vi "uEye_Binning_and_Subsampling.vi"() -> ()   [LabVIEW 2010]
uses:
  C:/Program Files (x86)/National Instruments/LabVIEW 2016/instr.lib/IDS/ueye.NET/uEyeDotNet.dll
  Program Files (x86)/National Instruments/LabVIEW 2016/instr.lib/IDS/ueye.NET/uEyeDotNet.dll
panel:
  out "Sensor Name":string
  out "Selected \nSubsampling Mode\nsupported":bool
  out "Selected \nBinning Mode \nsupported":bool
  in  "Vertical":i32(ring) items=["1x"=0, "2x"=1, "3x"=16, "4x"=4, "5x"=64, "6x"=256, "8x"=1024, "16x"=4096]
  in  "Horizontal":i32(ring) items=["1x"=0, "2x"=2, "3x"=32, "4x"=8, "5x"=128, "6x"=512, "8x"=2048, "16x"=8192]
  in  "Vertical":i32(ring) items=["1x"=0, "2x"=1, "3x"=16, "4x"=4, "5x"=64, "6x"=256, "8x"=1024, "16x"=4096]
  in  "Horizontal":i32(ring) items=["1x"=0, "2x"=2, "3x"=32, "4x"=8, "5x"=128, "6x"=512, "8x"=2048, "16x"=8192]
  out "Image":picture
  in  "Camera ID":i32 min=0 max=255
  out "Serial Number":string
  out "Height":i32=8
  out "Width":i32=8
  out "Bits/Pixel":i32=8
  out "Error Out":errorcluster caption="error"
  in  "Exit Camera":bool
  in  "Init Camera":bool
  # "Binning"
  # "Subsampling"
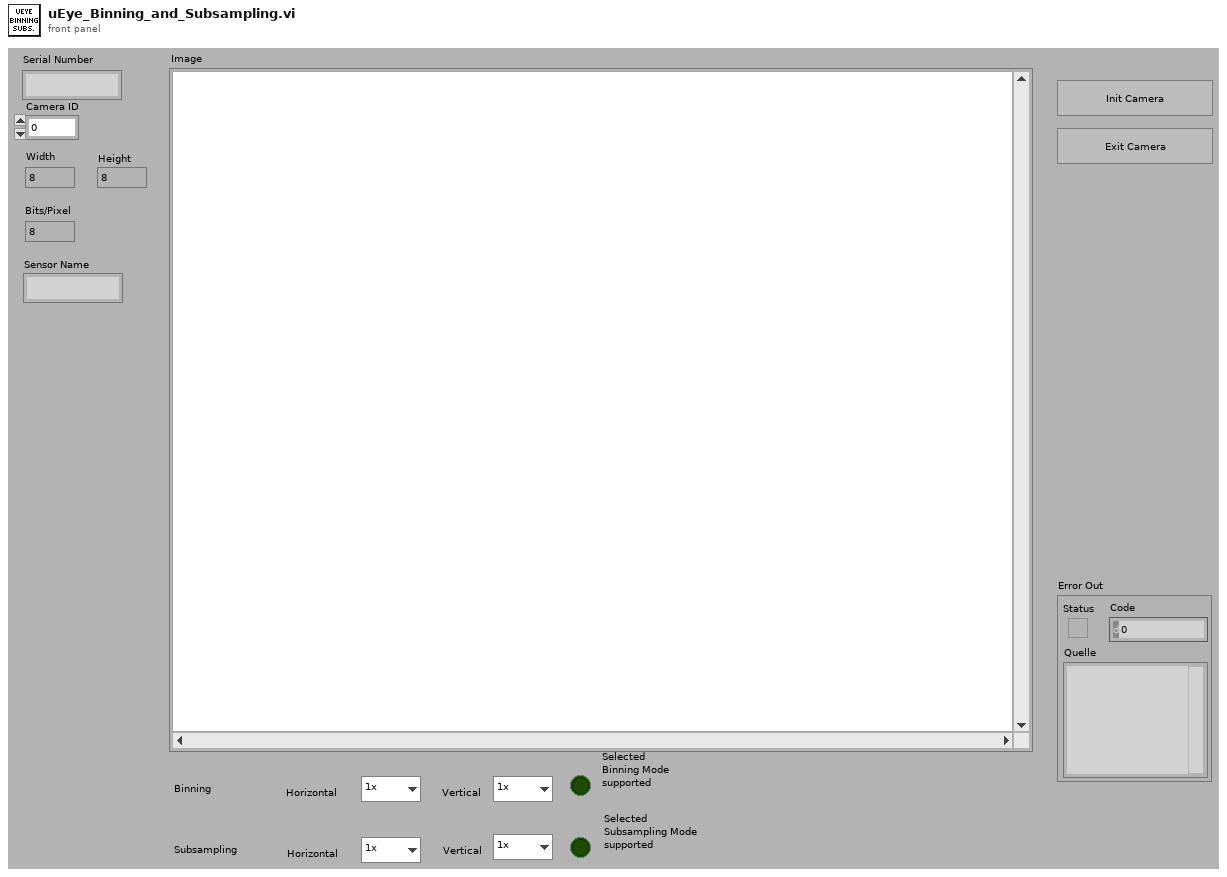
[diagram p1: front panel]
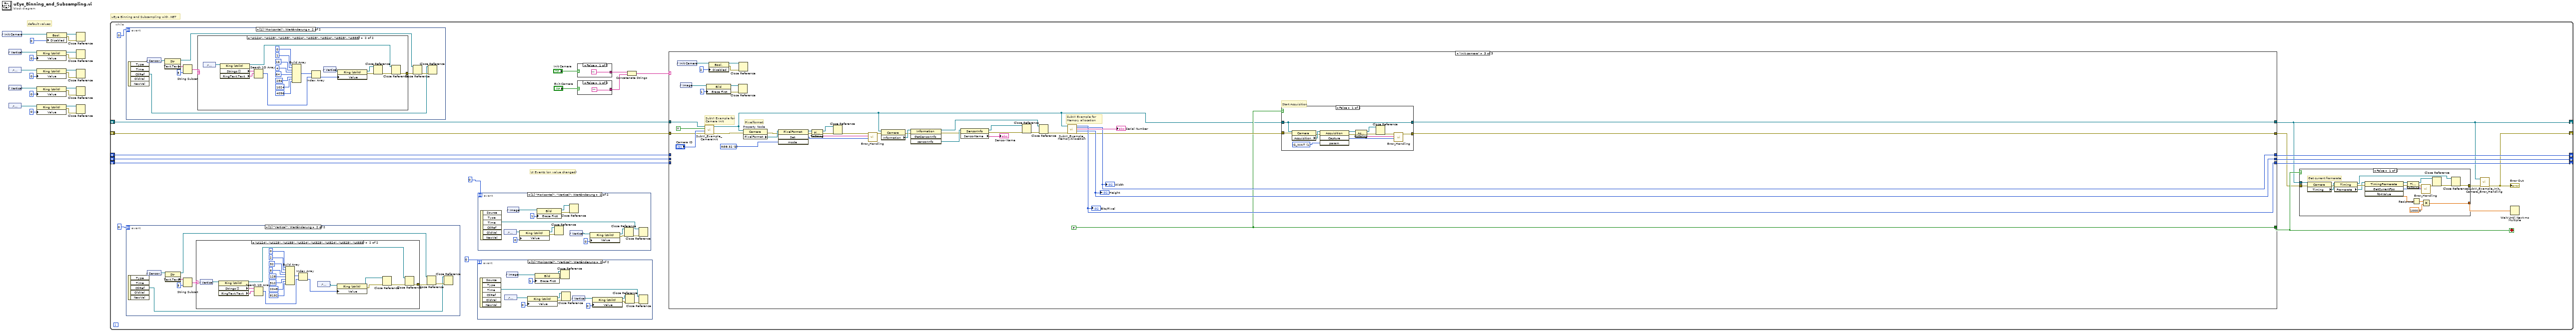
[diagram p0: block diagram]
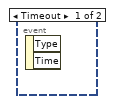
[diagram p2: hidden frame]
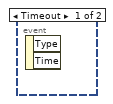
[diagram p4: hidden frame]
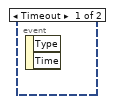
[diagram p6: hidden frame]
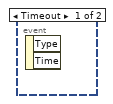
[diagram p7: hidden frame]
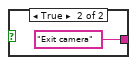
[diagram p8: hidden frame]
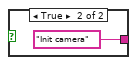
[diagram p9: hidden frame]
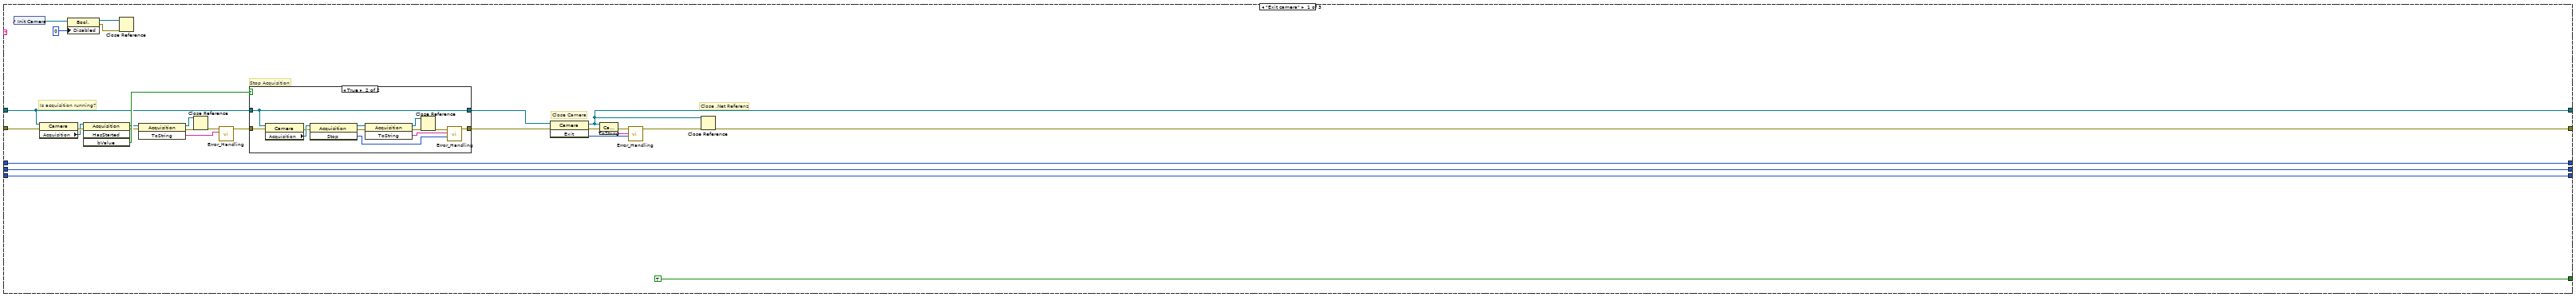
[diagram p10: hidden frame]
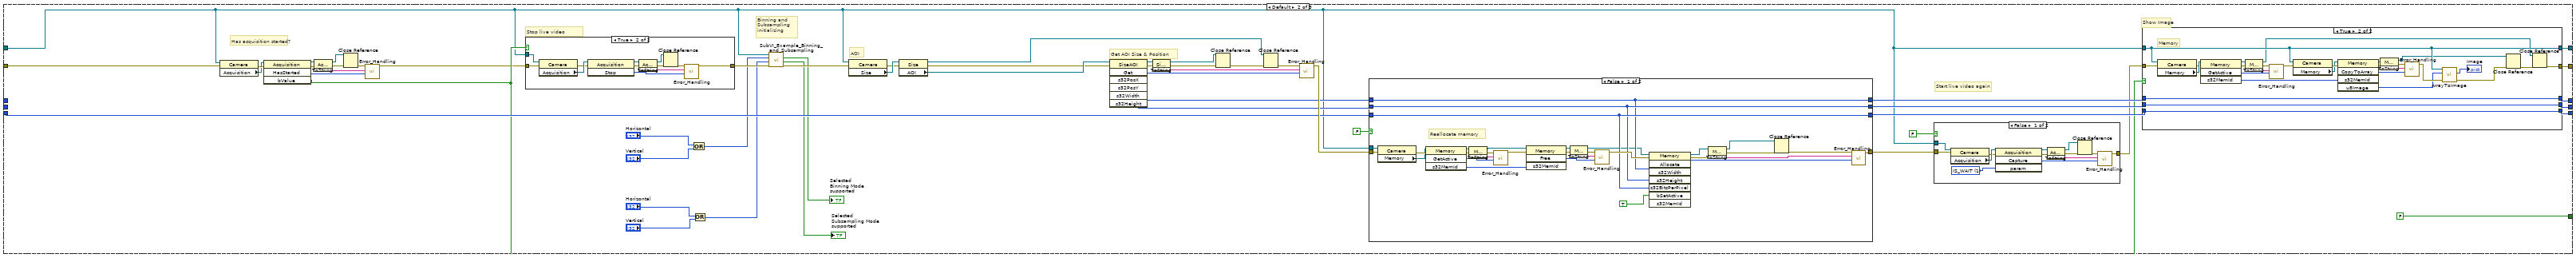
[diagram p12: hidden frame]
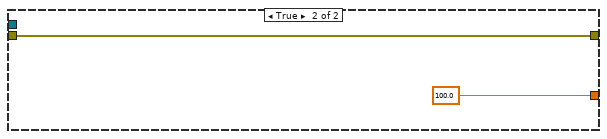
[diagram p18: hidden frame]
diagram:
  # "default values"
  # "uEye Binning and Subsampling with .NET"
  n1 = control-ref of="Init Camera"() -> (w19:refnum<vi>)
  n2 = control-ref of="Vertical"() -> (w11:refnum<vi>)
  n3 = control-ref of="Horizontal"() -> (w12:refnum<vi>)
  n4 = control-ref of="Vertical"() -> (w13:refnum<vi>)
  n5 = control-ref of="Horizontal"() -> (w14:refnum<vi>)
  n6 = property class="Ring (strikt)"(reference=w11, "Value"=0) -> (reference out=w8:refnum<vi>, error out=w7:errorcluster)  [unwired: 1 in]
  n7 = property class="Ring (strikt)"(reference=w12, "Value"=0) -> (reference out=w6:refnum<vi>, error out=w5:errorcluster)  [unwired: 1 in]
  n8 = property class="Ring (strikt)"(reference=w13, "Value"=0) -> (reference out=w4:refnum<vi>, error out=w3:errorcluster)  [unwired: 1 in]
  n9 = property class="Ring (strikt)"(reference=w14, "Value"=0) -> (reference out=w2:refnum<vi>, error out=w1:errorcluster)  [unwired: 1 in]
  n10 = property class="Bool."(reference=w19, "Disabled"=u8 0 ("Deaktiviert")) -> (reference out=w10:refnum<vi>, error out=w9:errorcluster)  [unwired: 1 in]
  n11 = Close Reference(reference=w10, error in (no error)=w9) -> ()  [unwired: 1 out]
  n12 = Close Reference(reference=w8, error in (no error)=w7) -> ()  [unwired: 1 out]
  n13 = Close Reference(reference=w6, error in (no error)=w5) -> ()  [unwired: 1 out]
  n14 = Close Reference(reference=w4, error in (no error)=w3) -> ()  [unwired: 1 out]
  n15 = Close Reference(reference=w2, error in (no error)=w1) -> ()  [unwired: 1 out]
  n16 = while {
    shift-right: [w28] -> _
    shift-left: _ -> [w38]
    shift-right: [w27] -> _
    shift-left: _ -> [w21]
    shift-right: [w35] -> _
    shift-left: _ -> [w34]
    shift-right: [w37] -> _
    shift-left: _ -> [w33]
    shift-right: [w36] -> _
    shift-left: _ -> [w32]
    stop <- w31 stop-if-true
    # "UI Events (on value changed)"
    n17 = event shown="[1] \"Horizontal\": Wertänderung" {
      selector: _ -> [_ _]
      dyn-events: _ -> [_ _]
      timeout: 0 -> [_ _]
      event Timeout {
        n18 = event-data() -> ()  [unwired: 1 in, 2 out]
      }
      event "Horizontal": Value Change {
        n19 = event-data() -> ("CtlRef"=w72:refnum<vi>)  [unwired: 1 in, 4 out]
        n20 = control-ref of="Sensor Name"() -> (w79:refnum<vi>)
        n21 = property class="Str"(reference=w79) -> (reference out=w74:refnum<vi>, "Text.Text"=w78:string)  [unwired: 1 in, 1 out]
        n22 = String Subset(string=w78, length (rest)=5 ("length (rest)")) -> (substring=w76:string)  [unwired: 1 in]
        n23 = case shown="\"UI124\", \"UI125\", \"UI155\", \"UI324\", \"UI325\", \"UI524\", \"UI525\", \"UI555\"" w76 {
          tunnel: [_ w80] -> w75
          frame "False", Default {
          }
          frame "UI124", "UI125", "UI155", "UI324", "UI325", "UI524", "UI525", "UI555" {
            n24 = control-ref of="Horizontal"() -> (w99:refnum<vi>)
            n25 = property class="Ring (strikt)"(reference=w99) -> (reference out=w81:refnum<vi>, "Strings []"=w97:string[], "RingText.Text"=w96:string)  [unwired: 1 in, 1 out]
            n26 = Search 1D Array(1D array=w97, element=w96) -> (index of element=w86:i32)  [unwired: 1 in]
            n27 = Build Array(0, 1, 16, 4, 64, 256, 1024, 4096) -> (w95:i32[])
            n28 = Index Array(array=w95, index=w86) -> (element=w85:i32)
            n29 = control-ref of="Vertical"() -> (w98:refnum<vi>)
            n30 = property class="Ring (strikt)"(reference=w98, "Value"=w85) -> (reference out=w83:refnum<vi>, error out=w84:errorcluster)  [unwired: 1 in]
            n31 = Close Reference(reference=w83, error in (no error)=w84) -> (error out=w82:errorcluster)
            n32 = Close Reference(reference=w81, error in (no error)=w82) -> (error out=w80:errorcluster)
          }
        }
        n33 = Close Reference(reference=w74, error in (no error)=w75) -> (error out=w73:errorcluster)
        n34 = Close Reference(reference=w72, error in (no error)=w73) -> ()  [unwired: 1 out]
      }
    }
    n35 = event shown="[1] \"Vertical\": Wertänderung" {
      selector: _ -> [_ _]
      dyn-events: _ -> [_ _]
      timeout: 0 -> [_ _]
      event Timeout {
        n36 = event-data() -> ()  [unwired: 1 in, 2 out]
      }
      event "Vertical": Value Change {
        n37 = event-data() -> ("CtlRef"=w44:refnum<vi>)  [unwired: 1 in, 4 out]
        n38 = control-ref of="Sensor Name"() -> (w49:refnum<vi>)
        n39 = property class="Str"(reference=w49) -> (reference out=w45:refnum<vi>, "Text.Text"=w51:string)  [unwired: 1 in, 1 out]
        n40 = String Subset(string=w51, length (rest)=5 ("length (rest)")) -> (substring=w48:string)  [unwired: 1 in]
        n41 = case shown="\"UI124\", \"UI125\", \"UI155\", \"UI324\", \"UI325\", \"UI524\", \"UI525\", \"UI555\"" w48 {
          tunnel: [_ w56] -> w46
          frame "False", Default {
          }
          frame "UI124", "UI125", "UI155", "UI324", "UI325", "UI524", "UI525", "UI555" {
            n42 = control-ref of="Vertical"() -> (w70:refnum<vi>)
            n43 = property class="Ring (strikt)"(reference=w70) -> (reference out=w55:refnum<vi>, "Strings []"=w69:string[], "RingText.Text"=w68:string)  [unwired: 1 in, 1 out]
            n44 = Search 1D Array(1D array=w69, element=w68) -> (index of element=w58:i32)  [unwired: 1 in]
            n45 = Build Array(0, 2, 32, 8, 128, 512, 2048, 8192) -> (w59:i32[])
            n46 = Index Array(array=w59, index=w58) -> (element=w57:i32)
            n47 = control-ref of="Horizontal"() -> (w71:refnum<vi>)
            n48 = property class="Ring (strikt)"(reference=w71, "Value"=w57) -> (reference out=w52:refnum<vi>, error out=w53:errorcluster)  [unwired: 1 in]
            n49 = Close Reference(reference=w52, error in (no error)=w53) -> (error out=w54:errorcluster)
            n50 = Close Reference(reference=w55, error in (no error)=w54) -> (error out=w56:errorcluster)
          }
        }
        n51 = Close Reference(reference=w45, error in (no error)=w46) -> (error out=w47:errorcluster)
        n52 = Close Reference(reference=w44, error in (no error)=w47) -> ()  [unwired: 1 out]
      }
    }
    n53 = event shown="[1] \"Horizontal\", \"Vertical\": Wertänderung" {
      selector: _ -> [_ _]
      dyn-events: _ -> [_ _]
      timeout: 0 -> [_ _]
      event Timeout {
        n54 = event-data() -> ()  [unwired: 1 in, 2 out]
      }
      event "Horizontal", "Vertical": Value Change {
        n55 = event-data() -> ("CtlRef"=w100:refnum<vi>)  [unwired: 1 in, 5 out]
        n56 = control-ref of="Horizontal"() -> (w110:refnum<vi>)
        n57 = control-ref of="Image"() -> (w112:refnum<vi>)
        n58 = property class="Ring (strikt)"(reference=w110, "Value"=0) -> (reference out=w104:refnum<vi>, error out=w105:errorcluster)  [unwired: 1 in]
        n59 = property class="Bild"(reference=w112, "Erase First"=u8 1 ("Zuerst löschen")) -> (reference out=w106:refnum<vi>, error out=w107:errorcluster)  [unwired: 1 in]
        n60 = Close Reference(reference=w106, error in (no error)=w107) -> ()  [unwired: 1 out]
        n61 = Close Reference(reference=w104, error in (no error)=w105) -> ()  [unwired: 1 out]
        n62 = control-ref of="Vertical"() -> (w108:refnum<vi>)
        n63 = property class="Ring (strikt)"(reference=w108, "Value"=0) -> (reference out=w102:refnum<vi>, error out=w103:errorcluster)  [unwired: 1 in]
        n64 = Close Reference(reference=w102, error in (no error)=w103) -> (error out=w101:errorcluster)
        n65 = Close Reference(reference=w100, error in (no error)=w101) -> ()  [unwired: 1 out]
      }
    }
    n66 = event shown="[1] \"Horizontal\", \"Vertical\": Wertänderung" {
      selector: _ -> [_ _]
      dyn-events: _ -> [_ _]
      timeout: 0 -> [_ _]
      event Timeout {
        n67 = event-data() -> ()  [unwired: 1 in, 2 out]
      }
      event "Horizontal", "Vertical": Value Change {
        n68 = event-data() -> ("CtlRef"=w114:refnum<vi>)  [unwired: 1 in, 5 out]
        n69 = control-ref of="Horizontal"() -> (w125:refnum<vi>)
        n70 = control-ref of="Image"() -> (w126:refnum<vi>)
        n71 = property class="Ring (strikt)"(reference=w125, "Value"=0) -> (reference out=w119:refnum<vi>, error out=w118:errorcluster)  [unwired: 1 in]
        n72 = property class="Bild"(reference=w126, "Erase First"=u8 1 ("Zuerst löschen")) -> (reference out=w121:refnum<vi>, error out=w120:errorcluster)  [unwired: 1 in]
        n73 = Close Reference(reference=w119, error in (no error)=w118) -> ()  [unwired: 1 out]
        n74 = Close Reference(reference=w121, error in (no error)=w120) -> ()  [unwired: 1 out]
        n75 = control-ref of="Vertical"() -> (w122:refnum<vi>)
        n76 = property class="Ring (strikt)"(reference=w122, "Value"=0) -> (reference out=w116:refnum<vi>, error out=w117:errorcluster)  [unwired: 1 in]
        n77 = Close Reference(reference=w116, error in (no error)=w117) -> (error out=w115:errorcluster)
        n78 = Close Reference(reference=w114, error in (no error)=w115) -> ()  [unwired: 1 out]
      }
    }
    n79 = case shown="False" "Init Camera" {
      tunnel: ["" "Init camera"] -> w42
      frame False {
      }
      frame True {
      }
    }
    n80 = case shown="False" "Exit Camera" {
      tunnel: ["" "Exit camera"] -> w39
      frame False {
      }
      frame True {
      }
    }
    n81 = Concatenate Strings(w42, w39) -> (w41:string)
    n82 = case shown="\"Init camera\"" w41 {
      tunnel: w21 -> [w141 w190 w358]
      tunnel: w38 -> [w142 w183 w357]
      tunnel: [w153 w217 w348] -> w27
      tunnel: [w154 w216 w347] -> w30
      tunnel: [w152 w220 w351] -> w35
      tunnel: [w151 w219 w352] -> w37
      tunnel: [w150 w218 w353] -> w36
      tunnel: w34 -> [w152 _ _]
      tunnel: w33 -> [w151 _ _]
      tunnel: w32 -> [w150 w206 _]
      tunnel: [TRUE FALSE w349] -> w31
      frame "Exit camera" {
        # "Close .Net Referenz"
        # "Is acquisition running?"
        # "Stop Acquisition"
        # "Close Camera"
        n83 = control-ref of="Init Camera"() -> (w137:refnum<vi>)
        n84 = property class="Camera"(reference=w141, error in=w142) -> (error out=w149:errorcluster, "Acquisition"=w148:refnum<k24>)  [unwired: 1 out]
        n85 = property class="Bool."(reference=w137, "Disabled"=u8 0 ("Deaktiviert")) -> (reference out=w132:refnum<vi>, error out=w133:errorcluster)  [unwired: 1 in]
        n86 = invoke class="Acquisition" method="HasStarted"(reference=w148, error in=w149) -> (reference out=w143:refnum<k24>, error out=w145:errorcluster, "bValue"=w147:bool)  [unwired: 2 in, 1 out]
        n87 = Close Reference(reference=w132, error in (no error)=w133) -> ()  [unwired: 1 out]
        n88 = invoke class="Acquisition" method="ToString"(reference=w143, error in=w145) -> (reference out=w134:refnum<k24>, error out=w136:errorcluster, "ToString"=w144:string)  [unwired: 1 in]
        n89 = Close Reference(reference=w134, error in (no error)=w136) -> (error out=w135:errorcluster)
        n90 = call "Error_Handling.vi"("Error String"=w144, "Error In"=w135) -> ("Error Out"=w146:errorcluster)  [unwired: 9 in]
        n91 = case shown="True" w147 {
          tunnel: [w162 w173] -> w139
          tunnel: w146 -> [w162 w174]
          tunnel: w141 -> [w161 w166]
          tunnel: [w161 w166] -> w140
          frame False {
          }
          frame True {
            n92 = property class="Camera"(reference=w166, error in=w174) -> (error out=w170:errorcluster, "Acquisition"=w171:refnum<k24>)  [unwired: 1 out]
            n93 = invoke class="Acquisition" method="Stop"(reference=w171, error in=w170) -> (reference out=w168:refnum<k24>, error out=w169:errorcluster, "Stop"=w167:i32)  [unwired: 1 in]
            n94 = invoke class="Acquisition" method="ToString"(reference=w168, error in=w169) -> (reference out=w163:refnum<k24>, error out=w165:errorcluster, "ToString"=w172:string)  [unwired: 1 in]
            n95 = Close Reference(reference=w163, error in (no error)=w165) -> (error out=w164:errorcluster)
            n96 = call "Error_Handling.vi"("Error Code"=w167, "Error String"=w172, "Error In"=w164) -> ("Error Out"=w173:errorcluster)  [unwired: 8 in]
          }
        }
        n97 = invoke class="Camera" method="Exit"(reference=w140, error in=w139) -> (reference out=w153:refnum<k24>, error out=w157:errorcluster, "Exit"=w156:i32)  [unwired: 1 in]
        n98 = invoke class="Camera" method="ToString"(reference=w153, error in=w157) -> (error out=w158:errorcluster, "ToString"=w159:string)  [unwired: 1 in, 1 out]
        n99 = call "Error_Handling.vi"("Error Code"=w156, "Error String"=w159, "Error In"=w158) -> ("Error Out"=w155:errorcluster)  [unwired: 8 in]
        n100 = Close Reference ("Close Referenz")(reference=w153, error in (no error)=w155) -> (error out=w154:errorcluster)
      }
      frame Default {
        # "Binning and Subsampling initializing"
        # "Start live video again"
        # "Stop live video"
        # "Get AOI Size & Position"
        # "AOI"
        # "Has acquisition started?"
        # "Show Image"
        n101 = property class="Camera"(reference=w190, error in=w183) -> (error out=w226:errorcluster, "Acquisition"=w225:refnum<k24>)  [unwired: 1 out]
        n102 = invoke class="Acquisition" method="HasStarted"(reference=w225, error in=w226) -> (reference out=w223:refnum<k24>, error out=w222:errorcluster, "HasStarted"=w221:i32, "bValue"=w202:bool)  [unwired: 2 in]
        n103 = invoke class="Acquisition" method="ToString"(reference=w223, error in=w222) -> (reference out=w175:refnum<k24>, error out=w177:errorcluster, "ToString"=w224:string)  [unwired: 1 in]
        n104 = Close Reference(reference=w175, error in (no error)=w177) -> (error out=w176:errorcluster)
        n105 = call "Error_Handling.vi"("Error Code"=w221, "Error String"=w224, "Error In"=w176) -> ("Error Out"=w185:errorcluster)  [unwired: 8 in]
        n106 = case shown="True" w202 {
          tunnel: [w228 w240] -> w192
          tunnel: w190 -> [_ w234]
          tunnel: w185 -> [w228 w233]
          frame False {
          }
          frame True {
            n107 = property class="Camera"(reference=w234, error in=w233) -> (error out=w232:errorcluster, "Acquisition"=w238:refnum<k24>)  [unwired: 1 out]
            n108 = invoke class="Acquisition" method="Stop"(reference=w238, error in=w232) -> (reference out=w236:refnum<k24>, error out=w237:errorcluster, "Stop"=w235:i32)  [unwired: 1 in]
            n109 = invoke class="Acquisition" method="ToString"(reference=w236, error in=w237) -> (reference out=w229:refnum<k24>, error out=w231:errorcluster, "ToString"=w239:string)  [unwired: 1 in]
            n110 = Close Reference(reference=w229, error in (no error)=w231) -> (error out=w230:errorcluster)
            n111 = call "Error_Handling.vi"("Error Code"=w235, "Error String"=w239, "Error In"=w230) -> ("Error Out"=w240:errorcluster)  [unwired: 8 in]
          }
        }
        n112 = Or(x="Horizontal", y="Vertical") -> (x .or. y?=w189:i32)
        n113 = Or(x="Horizontal", y="Vertical") -> (x .or. y?=w188:i32)
        n114 = call "SubVI_Example_Binning_and_Subsampling.vi"("Error In"=w192, "Subsampling Mode"=w188, "Binning Mode"=w189, ".NET (Reference)"=w190) -> ("Error Out"=w191:errorcluster, "Subsampling mode supported"=→"Selected \nSubsampling Mode\nsupported":bool, "Binning mode supported"=→"Selected \nBinning Mode \nsupported":bool)  [unwired: 5 in]
        n115 = property class="Camera"(reference=w190, error in=w191) -> (error out=w214:errorcluster, "Size"=w215:refnum<k24>)  [unwired: 1 out]
        n116 = property class="Size"(reference=w215, error in=w214) -> (reference out=w178:refnum<k24>, error out=w184:errorcluster, "AOI"=w193:refnum<k24>)
        n117 = invoke class="SizeAOI" method="Get"(reference=w193, error in=w184) -> (reference out=w212:refnum<k24>, error out=w211:errorcluster, "Get"=w210:i32, "s32Width"=w208:i32, "s32Height"=w207:i32)  [unwired: 5 in, 2 out]
        n118 = invoke class="SizeAOI" method="ToString"(reference=w212, error in=w211) -> (reference out=w181:refnum<k24>, error out=w182:errorcluster, "ToString"=w213:string)  [unwired: 1 in]
        n119 = Close Reference(reference=w181, error in (no error)=w182) -> (error out=w180:errorcluster)
        n120 = Close Reference(reference=w178, error in (no error)=w180) -> (error out=w179:errorcluster)
        n121 = call "Error_Handling.vi"("Error Code"=w210, "Error String"=w213, "Error In"=w179) -> ("Error Out"=w209:errorcluster)  [unwired: 8 in]
        n122 = case shown="False" FALSE {
          tunnel: w209 -> [w266 w286]
          tunnel: w208 -> [w262 w289]
          tunnel: w207 -> [w263 w288]
          tunnel: w206 -> [w264 w287]
          tunnel: [w265 w286] -> w201
          tunnel: [w264 w287] -> w205
          tunnel: [w263 w288] -> w204
          tunnel: [w262 w289] -> w203
          tunnel: w190 -> [w261 _]
          frame False {
            # "Reallocate memory"
            n123 = property class="Camera"(reference=w261, error in=w266) -> (error out=w268:errorcluster, "Memory"=w259:refnum<k24>)  [unwired: 1 out]
            n124 = invoke class="Memory" method="GetActive"(reference=w259, error in=w268) -> (reference out=w273:refnum<k24>, error out=w272:errorcluster, "GetActive"=w271:i32, "s32MemId"=w270:i32)  [unwired: 2 in]
            n125 = invoke class="Memory" method="ToString"(reference=w273, error in=w272) -> (reference out=w258:refnum<k24>, error out=w274:errorcluster, "ToString"=w275:string)  [unwired: 1 in]
            n126 = call "Error_Handling.vi"("Error Code"=w271, "Error String"=w275, "Error In"=w274) -> ("Error Out"=w269:errorcluster)  [unwired: 8 in]
            n127 = invoke class="Memory" method="Free"(reference=w258, error in=w269, "s32MemId"=w270) -> (reference out=w278:refnum<k24>, error out=w277:errorcluster, "Free"=w276:i32)  [unwired: 1 in, 1 out]
            n128 = invoke class="Memory" method="ToString"(reference=w278, error in=w277) -> (reference out=w255:refnum<k24>, error out=w279:errorcluster, "ToString"=w280:string)  [unwired: 1 in]
            n129 = call "Error_Handling.vi"("Error Code"=w276, "Error String"=w280, "Error In"=w279) -> ("Error Out"=w267:errorcluster)  [unwired: 8 in]
            n130 = invoke class="Memory" method="Allocate"(reference=w255, error in=w267, "s32Width"=w262, "s32Height"=w263, "s32BitsPerPixel"=w264, "bSetActive"=TRUE) -> (reference out=w284:refnum<k24>, error out=w283:errorcluster, "Allocate"=w282:i32)  [unwired: 2 in, 5 out]
            n131 = invoke class="Memory" method="ToString"(reference=w284, error in=w283) -> (reference out=w256:refnum<k24>, error out=w257:errorcluster, "ToString"=w285:string)  [unwired: 1 in]
            n132 = Close Reference(reference=w256, error in (no error)=w257) -> (error out=w260:errorcluster)
            n133 = call "Error_Handling.vi"("Error Code"=w282, "Error String"=w285, "Error In"=w260) -> ("Error Out"=w265:errorcluster)  [unwired: 8 in]
          }
          frame True {
          }
        }
        n134 = case shown="False" FALSE {
          tunnel: [w246 w254] -> w199
          tunnel: w201 -> [w251 w254]
          tunnel: w190 -> [w250 _]
          frame False {
            w244 = 1 items=["IS_DONT_WAIT", "IS_WAIT"] ("Wait")
            n135 = property class="Camera"(reference=w250, error in=w251) -> (error out=w252:errorcluster, "Acquisition"=w253:refnum<k24>)  [unwired: 1 out]
            n136 = invoke class="Acquisition" method="Capture"(reference=w253, error in=w252, "param"=w244) -> (reference out=w247:refnum<k24>, error out=w248:errorcluster, "Capture"=w245:i32)  [unwired: 1 in, 1 out]
            n137 = invoke class="Acquisition" method="ToString"(reference=w247, error in=w248) -> (reference out=w241:refnum<k24>, error out=w243:errorcluster, "ToString"=w249:string)  [unwired: 1 in]
            n138 = Close Reference(reference=w241, error in (no error)=w243) -> (error out=w242:errorcluster)
            n139 = call "Error_Handling.vi"("Error Code"=w245, "Error String"=w249, "Error In"=w242) -> ("Error Out"=w246:errorcluster)  [unwired: 8 in]
          }
          frame True {
          }
        }
        n140 = case shown="True" w202 {
          tunnel: [w294 w299] -> w216
          tunnel: w199 -> [w294 w304]
          tunnel: w190 -> [w293 w300]
          tunnel: [w293 w300] -> w217
          tunnel: w203 -> [w292 w307]
          tunnel: w204 -> [w291 w306]
          tunnel: w205 -> [w290 w305]
          tunnel: [w292 w307] -> w220
          tunnel: [w291 w306] -> w219
          tunnel: [w290 w305] -> w218
          frame False {
          }
          frame True {
            # "Memory"
            n141 = property class="Camera"(reference=w300, error in=w304) -> (error out=w309:errorcluster, "Memory"=w310:refnum<k24>)  [unwired: 1 out]
            n142 = invoke class="Memory" method="GetActive"(reference=w310, error in=w309) -> (reference out=w316:refnum<k24>, error out=w315:errorcluster, "GetActive"=w317:i32, "s32MemId"=w308:i32)  [unwired: 2 in]
            n143 = invoke class="Memory" method="ToString"(reference=w316, error in=w315) -> (reference out=w298:refnum<k24>, error out=w313:errorcluster, "ToString"=w314:string)  [unwired: 1 in]
            n144 = call "Error_Handling.vi"("Error Code"=w317, "Error String"=w314, "Error In"=w313) -> ("Error Out"=w318:errorcluster)  [unwired: 8 in]
            n145 = property class="Camera"(reference=w300, error in=w318) -> (error out=w312:errorcluster, "Memory"=w311:refnum<k24>)  [unwired: 1 out]
            n146 = invoke class="Memory" method="CopyToArray"(reference=w311, error in=w312, "s32MemId"=w308) -> (reference out=w321:refnum<k24>, error out=w322:errorcluster, "CopyToArray"=w323:i32, "u8Image"=w301:u8[])  [unwired: 2 in, 1 out]
            n147 = invoke class="Memory" method="ToString"(reference=w321, error in=w322) -> (reference out=w295:refnum<k24>, error out=w319:errorcluster, "ToString"=w320:string)  [unwired: 1 in]
            n148 = call "Error_Handling.vi"("Error Code"=w323, "Error String"=w320, "Error In"=w319) -> ("Error Out"=w302:errorcluster)  [unwired: 8 in]
            n149 = call "ArrayToImage.vi"("Error In"=w302, "InArray"=w301, ".NET (Reference)"=w300) -> ("Error Out"=w296:errorcluster, "Image"=→"Image":picture)  [unwired: 7 in]
            n150 = Close Reference(reference=w295, error in (no error)=w296) -> (error out=w297:errorcluster)
            n151 = Close Reference(reference=w298, error in (no error)=w297) -> (error out=w299:errorcluster)
          }
        }
      }
      frame "Init camera" {
        w349 = FALSE
        w366 = 0 items=["RGB 32"=0, "RGB 24"=1, "Y8 Monochrom"=6] ("Mode")
        # "Start Acquisition"
        # "SubVI Example for \nMemory allocation"
        # "SubVI Example for \nCamera Init"
        # "Pixelformat"
        n152 = control-ref of="Init Camera"() -> (w346:refnum<vi>)
        n153 = control-ref of="Image"() -> (w343:refnum<vi>)
        n154 = call "SubVI_Example_CameraInit.vi"("Error In"=w357, "Camera ID"="Camera ID", "Init Camera Flag"=TRUE, ".NET (Reference)"=w358) -> ("Error Out"=w363:errorcluster, ".NET (Reference)"=w340:refnum<k24>)  [unwired: 6 in]
        n155 = property class="Bild"(reference=w343, "Erase First"=u8 1 ("Zuerst löschen")) -> (reference out=w325:refnum<vi>, error out=w326:errorcluster)  [unwired: 1 in]
        n156 = property class="Bool."(reference=w346, "Disabled"=u8 2 ("Deaktiviert")) -> (reference out=w324:refnum<vi>, error out=w327:errorcluster)  [unwired: 1 in]
        n157 = Close Reference(reference=w325, error in (no error)=w326) -> ()  [unwired: 1 out]
        n158 = Close Reference(reference=w324, error in (no error)=w327) -> ()  [unwired: 1 out]
        n159 = property on="Property Node" class="Camera"(reference=w340, error in=w363) -> (error out=w364:errorcluster, "PixelFormat"=w365:refnum<k24>)  [unwired: 1 out]
        n160 = invoke class="PixelFormat" method="Set"(reference=w365, error in=w364, "mode"=w366) -> (reference out=w361:refnum<k24>, error out=w355:errorcluster, "Set"=w360:i32)  [unwired: 1 in, 1 out]
        n161 = invoke class="PixelFormat" method="ToString"(reference=w361, error in=w355) -> (reference out=w333:refnum<k24>, error out=w335:errorcluster, "ToString"=w362:string)  [unwired: 1 in]
        n162 = Close Reference(reference=w333, error in (no error)=w335) -> (error out=w334:errorcluster)
        n163 = call "Error_Handling.vi"("Error Code"=w360, "Error String"=w362, "Error In"=w334) -> ("Error Out"=w341:errorcluster)  [unwired: 8 in]
        n164 = property class="Camera"(reference=w340, error in=w341) -> (error out=w339:errorcluster, "Information"=w342:refnum<k24>)  [unwired: 1 out]
        n165 = invoke class="Information" method="GetSensorInfo"(reference=w342, error in=w339) -> (reference out=w328:refnum<k24>, error out=w337:errorcluster, "sensorInfo"=w338:refnum<k24>)  [unwired: 2 in, 1 out]
        n166 = property class="SensorInfo"(reference=w338, error in=w337) -> (reference out=w331:refnum<k24>, error out=w332:errorcluster, "SensorName"=→"Sensor Name":string)
        n167 = Close Reference(reference=w331, error in (no error)=w332) -> (error out=w330:errorcluster)
        n168 = Close Reference(reference=w328, error in (no error)=w330) -> (error out=w329:errorcluster)
        n169 = call "SubVI_Example_MemoryAllocation.vi"(".NET (Reference)"=w340, "Error In"=w329) -> ("Bits/Pixel 2"=w353:i32, "Width"=w351:i32, "Serial Number"=→"Serial Number":string, "Height"=w352:i32, "Error Out"=w350:errorcluster)  [unwired: 13 in]
        "Bits/Pixel" <- w353
        "Width" <- w351
        "Height" <- w352
        n170 = case shown="False" w349 {
          tunnel: [w372 w381] -> w347
          tunnel: w350 -> [w377 w381]
          tunnel: w340 -> [w376 w380]
          tunnel: [w376 w380] -> w348
          frame False {
            w370 = 1 items=["IS_DONT_WAIT", "IS_WAIT"] ("Wait")
            n171 = property class="Camera"(reference=w376, error in=w377) -> (error out=w378:errorcluster, "Acquisition"=w379:refnum<k24>)  [unwired: 1 out]
            n172 = invoke class="Acquisition" method="Capture"(reference=w379, error in=w378, "param"=w370) -> (reference out=w373:refnum<k24>, error out=w374:errorcluster, "Capture"=w371:i32)  [unwired: 1 in, 1 out]
            n173 = invoke class="Acquisition" method="ToString"(reference=w373, error in=w374) -> (reference out=w367:refnum<k24>, error out=w369:errorcluster, "ToString"=w375:string)  [unwired: 1 in]
            n174 = Close Reference(reference=w367, error in (no error)=w369) -> (error out=w368:errorcluster)
            n175 = call "Error_Handling.vi"("Error Code"=w371, "Error String"=w375, "Error In"=w368) -> ("Error Out"=w372:errorcluster)  [unwired: 8 in]
          }
          frame True {
          }
        }
      }
    }
    n176 = case shown="False" w31 {
      tunnel: [w395 100.0] -> w43
      tunnel: w27 -> [w394 _]
      tunnel: w30 -> [w393 w403]
      tunnel: [w383 w403] -> w29
      frame False {
        # "Get current framerate"
        n177 = property class="Camera"(reference=w394, error in=w393) -> (error out=w397:errorcluster, "Timing"=w396:refnum<k24>)  [unwired: 1 out]
        n178 = property class="Timing"(reference=w396, error in=w397) -> (reference out=w382:refnum<k24>, error out=w399:errorcluster, "Framerate"=w385:refnum<k24>)
        n179 = invoke class="TimingFramerate" method="GetCurrentFps"(reference=w385, error in=w399) -> (reference out=w388:refnum<k24>, error out=w389:errorcluster, "GetCurrentFps"=w390:i32, "f64Value"=w398:dbl)  [unwired: 2 in]
        n180 = invoke class="TimingFramerate" method="ToString"(reference=w388, error in=w389) -> (reference out=w386:refnum<k24>, error out=w392:errorcluster, "ToString"=w391:string)  [unwired: 1 in]
        n181 = Reciprocal(x=w398) -> (1/x=w401:dbl)
        n182 = call "Error_Handling.vi"("Error Code"=w390, "Error String"=w391, "Error In"=w392) -> ("Error Out"=w387:errorcluster)  [unwired: 8 in]
        n183 = Multiply(x=w401, y=1000.0) -> (x*y=w395:dbl)
        n184 = Close Reference(reference=w386, error in (no error)=w387) -> (error out=w384:errorcluster)
        n185 = Close Reference(reference=w382, error in (no error)=w384) -> (error out=w383:errorcluster)
      }
      frame True {
      }
    }
    n186 = call "SubVI_Example_Init_Camera_Error_Handling.vi"("Error In"=w29, ".NET (Reference)"=w27) -> ("Error Out"=w28:errorcluster)  [unwired: 9 in]
    "Error Out" <- w28
    n187 = Wait Until Next ms Multiple(millisecond multiple=w43) -> ()  [unwired: 1 out]
  }
